vi "Move Relative.vi"(8 "Move":refnum<class "Point.lvclass">, 11 "Point":refnum<class "Point.lvclass">) -> (3 "New Point":refnum<class "Point.lvclass">)   [LabVIEW 2021, in "Picture2D.lvlib" / "Shape.lvclass"]
uses:
  Shape.lvclass
  Point/Point.lvclass
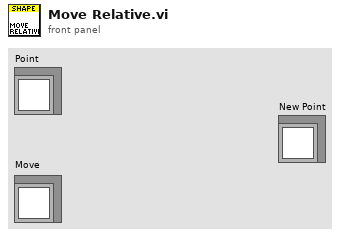
[diagram p1: front panel]
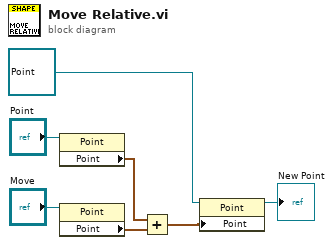
[diagram p0: block diagram]
diagram:
  n1 = property class="Point"(reference="Point") -> ("Point"=w3:cluster{"x":i16, "y":i16})  [unwired: 1 in, 2 out]
  n2 = property class="Point"(reference="Move") -> ("Point"=w2:cluster{"x":i16, "y":i16})  [unwired: 1 in, 2 out]
  n3 = Add(x=w3, y=w2) -> (x+y=w1:cluster{"x":i16, "y":i16})
  n4 = property class="Point"(reference=refnum<class "Point.lvclass"> refnum, "Point"=w1) -> (reference out=→"New Point":refnum<class "Point.lvclass">)  [unwired: 1 in, 1 out]
